vi "RCServoSetMaxPulseWidth.vi"(0 "error in (no error)":errorcluster, 2 "Max Pulse Width":dbl, 3 "Device In":u64) -> (7 "error out":errorcluster, 10 "Device Out":u64)   [LabVIEW 2020, in "Phidget RC Servo.lvlib"]
doc: "${MaxPulseWidth:Header}"
uses:
  <instrlib>/Phidgets/Phidget RC Servo/Phidget RC Servo.lvlib
  <instrlib>/Phidgets/Phidget Common/Phidget Common.lvlib
  phidget22.dll
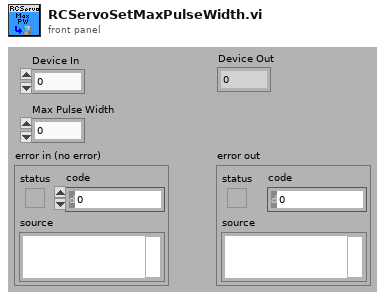
[diagram p1: front panel]
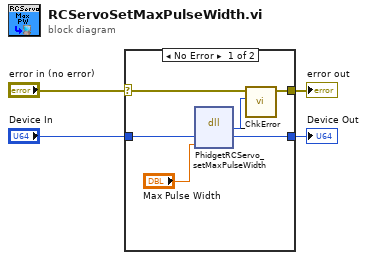
[diagram p0: block diagram]
diagram:
  n1 = case shown="No Error" "error in (no error)" {
    selector: "error in (no error)" -> [w7 w12]
    tunnel: [w6 w12] -> w3
    tunnel: "Device In" -> [w9 w11]
    tunnel: [w8 w11] -> w1
    frame No Error {
      n2 = dll-call lib="phidget22.*" fn="PhidgetRCServo_setMaxPulseWidth"("phid"=w9, "interval"="Max Pulse Width") -> ("return type"=w5:i32, "phid"=w8:u64)  [unwired: 4 in, 2 out]
      n3 = call <instrlib>:"_ChkError.vi"("Return Code"=w5, "error in (no error)"=w7) -> ("error out"=w6:errorcluster)  [unwired: 9 in]
    }
    frame Error {
    }
  }
  "error out" <- w3
  "Device Out" <- w1
